vi "G4SubTemplate_Simple_4x4x4_ReadProperty.vi"(8 "error in (no error)":errorcluster, 11 "reference in":refnum<class "G4SubTemplate_Simple_4x4x4.lvclass">) -> (0 "error out":errorcluster, 2 "property":dbl, 3 "reference in":refnum<class "G4SubTemplate_Simple_4x4x4.lvclass">)   [LabVIEW 2014]
uses:
  <resource>/Framework/Providers/Open_GDS/ClassProviders/Provider_EndevoGOOP400/Templates/G4SubTemplate_Simple_4x4x4/G4SubTemplate_Simple_4x4x4.lvclass
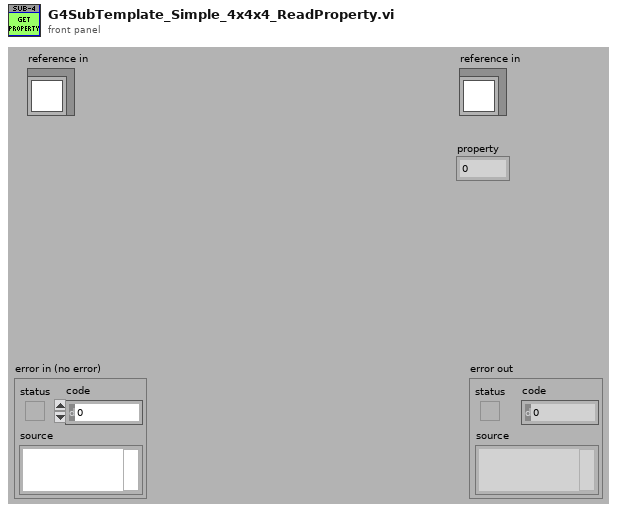
[diagram p1: front panel]
types:
  T1 = typedef "G4SubTemplate_Simple_4x4x4.lvclass/ObjectAttributes.ctl" = cluster{"Attribute1":dbl}
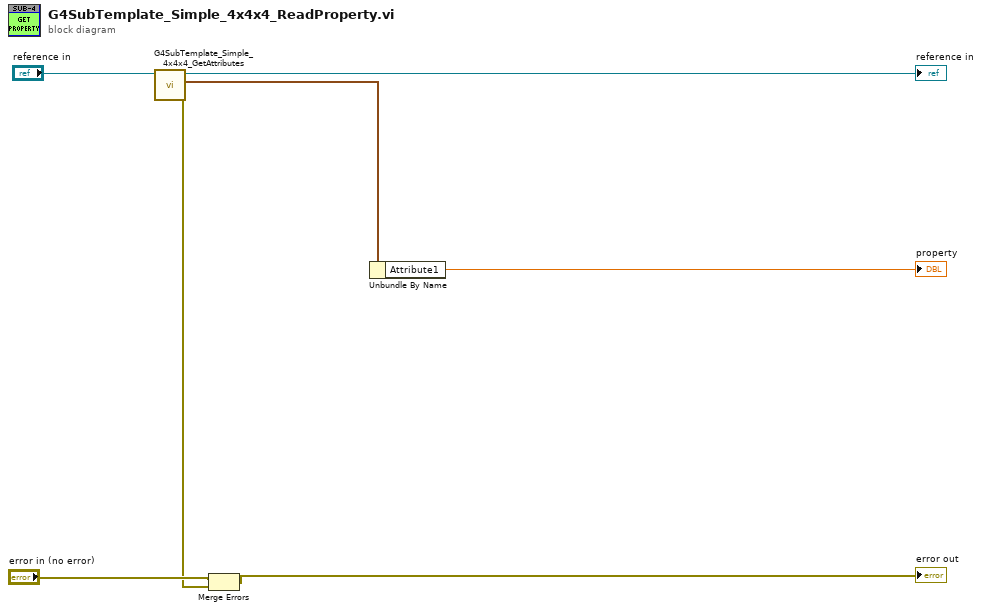
[diagram p0: block diagram]
diagram:
  n1 = call <resource>:"G4SubTemplate_Simple_4x4x4_GetAttributes.vi"("reference in"="reference in") -> ("error out"=w2:errorcluster, "Data"=w4:T1, "reference out"=→"reference in":refnum<class "G4SubTemplate_Simple_4x4x4.lvclass">)  [unwired: 7 in, 1 out]
  n2 = Merge Errors("error in (no error)", w2) -> (→"error out":errorcluster)
  n3 = Unbundle By Name(w4) -> ("Attribute1"=→"property":dbl)
